vi "TDMS2TDMCheckPaths.vi"(8 "error in (no error)":errorcluster, 10 "New TDM Path In":path, 11 "TDMS Path In":path) -> (0 "error out":errorcluster, 2 "New TDM File Out":path, 3 "TDMS File Out":path)   [LabVIEW 2017]
doc: "This VI checks to see if valid paths have been entered for the source and target files. If not, a dialog prompts for a valid file path. If only a directory is given for the target path, then a default filename is created in that directory using the source filename and the target extension."
uses:
  <vilib>/Utility/tdmsutil.llb/TDMSFileViewerLocalizedText.vi
  Instance           1 26Saved   TDMS2TDMCheckPaths .vi
  Instance           2 26Saved   TDMS2TDMCheckPaths .vi
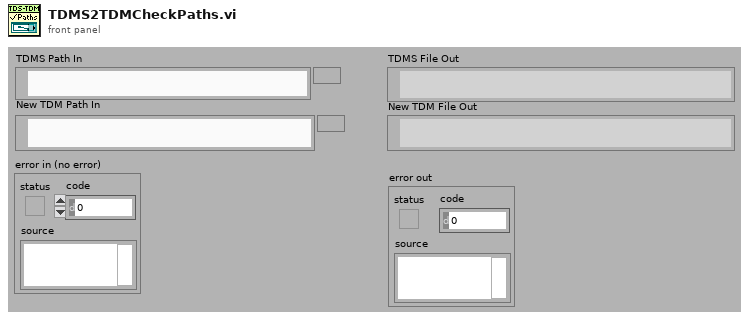
[diagram p1: front panel]
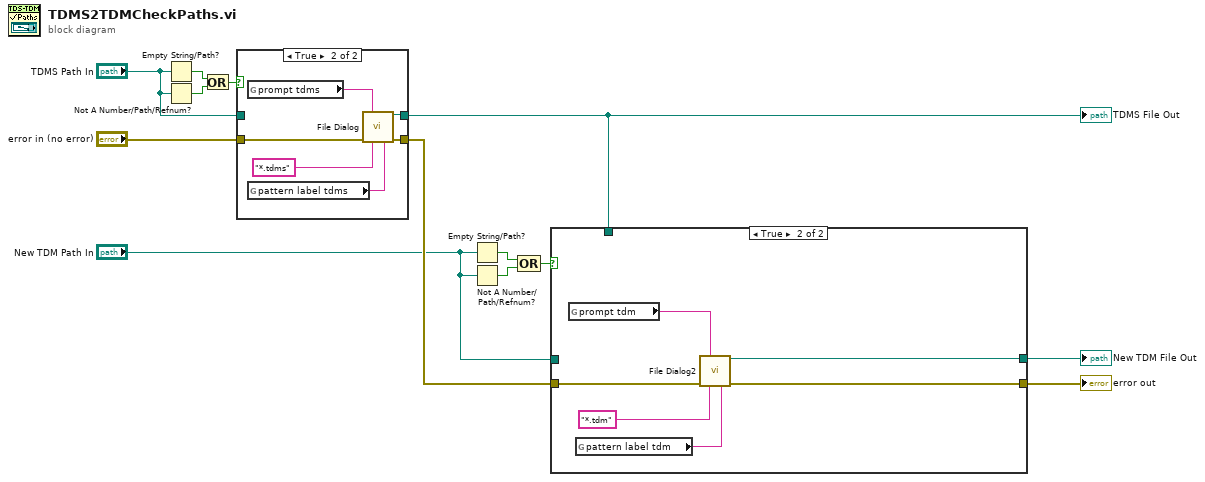
[diagram p0: block diagram]
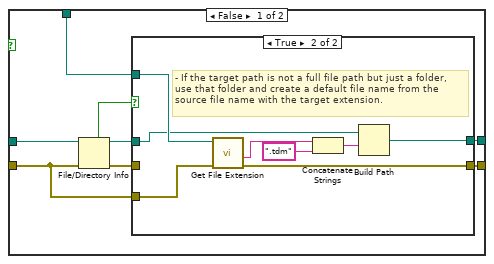
[diagram p2: hidden frame]
diagram:
  n1 = Empty String/Path?(string/path="TDMS Path In") -> (empty?=w12:bool)
  n2 = Not A Number/Path/Refnum?(number/path/refnum="TDMS Path In") -> (NaN/Path/Refnum?=w11:bool)
  n3 = Or(x=w12, y=w11) -> (x .or. y?=w10:bool)
  n4 = case shown="True" w10 {
    tunnel: "TDMS Path In" -> [w15 _]
    tunnel: [w15 w21] -> w1
    tunnel: [w14 w20] -> w5
    tunnel: "error in (no error)" -> [w14 w19]
    frame False {
    }
    frame True {
      n5 = global read "TDMSFileViewerLocalizedText.vi" "prompt tdms"() -> (w18:string)
      n6 = global read "TDMSFileViewerLocalizedText.vi" "pattern label tdms"() -> (w16:string)
      n7 = call "File Dialog"("prompt"=w18, "error in"=w19, "pattern (all files)"="*.tdms" ("pattern label"), "pattern label"=w16) -> ("selected path"=w21:path, "error out"=w20:errorcluster)  [unwired: 8 in, 2 out]
    }
  }
  "TDMS File Out" <- w1
  n8 = Empty String/Path?(string/path="New TDM Path In") -> (empty?=w6:bool)
  n9 = Not A Number/Path/Refnum?(number/path/refnum="New TDM Path In") -> (NaN/Path/Refnum?=w7:bool)
  n10 = Compound Arithmetic op=OR(w6, w7) -> (w8:bool)
  n11 = case shown="True" w8 {
    tunnel: "New TDM Path In" -> [w26 _]
    tunnel: [w23 w45] -> w2
    tunnel: w5 -> [w25 w44]
    tunnel: [w24 w43] -> w3
    tunnel: w1 -> [w22 _]
    frame False {
      n12 = File/Directory Info(path=w26, error in=w25) -> (path out=w28:path, directory=w27:bool, error out=w29:errorcluster)  [unwired: 4 out]
      n13 = case shown="True" w27 {
        tunnel: [w31 w36] -> w23
        tunnel: w28 -> [w31 w37]
        tunnel: w25 -> [w30 w38]
        tunnel: w22 -> [_ w39]
        tunnel: [w30 w35] -> w24
        tunnel: w29 -> [_ _]
        frame False {
        }
        frame True {
          # "- If the target path is not a full file path but just a folder,\nuse that folder and create a default file name from the\nsource file name with the target extension."
          n14 = call <vilib>:"Get File Extension.vi"("error in (no error)"=w38, "file"=w39) -> ("error out"=w35:errorcluster, "filename without extension"=w34:string)  [unwired: 5 in, 3 out]
          n15 = Concatenate Strings(w34, ".tdm") -> (w33:string)
          n16 = Build Path(base path=w37, name or relative path=w33) -> (appended path=w36:path)
        }
      }
    }
    frame True {
      n17 = global read "TDMSFileViewerLocalizedText.vi" "prompt tdm"() -> (w42:string)
      n18 = global read "TDMSFileViewerLocalizedText.vi" "pattern label tdm"() -> (w41:string)
      n19 = call "File Dialog2"("prompt"=w42, "error in"=w44, "pattern (all files)"="*.tdm" ("pattern label"), "pattern label"=w41) -> ("selected path"=w45:path, "error out"=w43:errorcluster)  [unwired: 8 in, 2 out]
    }
  }
  "New TDM File Out" <- w2
  "error out" <- w3
